vi "SEA_9811_Init.vi"(7 "Run?":bool=TRUE, 8 "error in":errorcluster, 9 "Transmit Channels Ref in":T1 format="%.0x", 10 "SEA9811_conf_cluster":T9={"FPGA resource name"="RIO0", "Rx ch conf (0..7)"=[{"Rx Channel Number (0..7)"=0, "Rx Label Filter"={"Label 00"=0, "Label 01"=0, "Label 02"=0, "Label 03"=0, "Label 04"=0, "Label 05"=0, "Label 06"=0, "Label 07"=0, "Label 08"=0, "Label 09"=0, "Label 10"=0, "Label 11"=0, "Label 12"=0, "Label 13"=0, "Label 14"=0, "Label 15"=0}, "Receiver Control Register (RCR)"={"RCR0: Data rate = ARINC 429 High-Speed (0) or Low-Speed (1)"=FALSE, "RCR1: not used"=FALSE, "RCR2: Label recognition for this channel enabled (1) or disabled (0)"=FALSE, "RCR3: Receiver channel disabled (1) or enabled (0)"=FALSE, "RCR4: Odd parity check for this channel enabled (1) or disabled (0"=FALSE, "RCR5: Receiver normal operation (1) or loopback mode (0)"=TRUE, "RCR6: Receiver Decoder disabled (0) or enabled (1) \n-> ARINC bits 10 and 9 must match RCR7 and RCR8"=FALSE, "RCR7: If receiver decoder is enabled (RCR6=1), \nthe ARINC bit 10 must match this bit"=FALSE, "RCR8: If receiver decoder is enabled (RCR6=1), \nthe ARINC bit 9 must match this bit"=FALSE, "RCR9: Label bit order for this channel non-reversed (1) \nor reversed (0)"=FALSE, "RCR10: not used"=FALSE, "RCR11: not used"=FALSE, "RCR12: not used"=FALSE, "RCR13: not used"=FALSE, "RCR14: not used"=FALSE, "RCR15: not used"=FALSE}}], "Transmitter Control Register (TCR)"={"TCR0: not used"=FALSE, "TCR1: not used"=FALSE, "TCR2: not used"=FALSE, "TCR3: Transmitter Parity Bit Enable: 32nd bit is parity (1) or data (0)"=FALSE, "TCR4: not used"=FALSE, "TCR5: not used"=FALSE, "TCR6: not used"=FALSE, "TCR7: not used"=FALSE, "TCR8: not used"=FALSE, "TCR9: Transmitter Parity Select: odd parity (0) or even parity (1)"=FALSE, "TCR10: Transmitter Data Rate: ARINC 429 high-speed (0) or low-speed (1)"=FALSE, "TCR11: ARINC Label Bit Order: label bit order reversed (0) or not reversed (1)"=FALSE, "TCR12: Disable Line Driver: normal operation (0) or transmitter disabled (1)"=FALSE, "TCR13: Tansmit whenever data is available in FIFO (1) or only start by instruction \"Enable Transmission\" (0)"=TRUE, "TCR14: not used"=FALSE, "TCR15: not used"=FALSE}, "Bitfile Path"=path ""}, 11 "Device Reference in":T1 format="%.0x") -> (0 "error out":errorcluster, 2 "SEA9811_RT_data out":T2 {"Tx"."Tx Refs (Data,Trig)"."Data Reference" format="%.0x"}, 3 "Device Reference out":T1 format="%.0x")   [LabVIEW 2015]
uses:
  Typdefs/SEA9811_RT_conf_cluster.ctl
  <vilib>/userdefined/High Color/nirio_resource_hc.ctl
  FPGA/SEA-9811_ReceiverAndTransmitter/SubVIs/SEA-9811_ReceiverAndTransmitter_RCR.ctl
  FPGA/SEA-9811_ReceiverAndTransmitter/SubVIs/SEA-9811_ReceiverAndTransmitter_TCR.ctl
  Typdefs/SEA9811_RT_data_cluster.ctl
  <userlib>/_FPGA Interface Advanced Tools/FPGA Interface Base/FPGA Interface Base.lvclass
  Typdefs/FPGA ref.ctl
  Typdefs/channel.ctl
  Typdefs/received word.ctl
  Typdefs/SEA9811_FPGA_FP_Addresses.ctl
  <vilib>/NI Veristand/Custom Device API/Block Data Reference.ctl
  <vilib>/NI Veristand/Custom Device API/Data Reference.ctl
  <vilib>/NI Veristand/Custom Device API/Custom Device Item Ref.ctl
  <vilib>/NI Veristand/Custom Device API/Data Access Type.ctl
  <vilib>/NI VeriStand/Custom Device API/Custom Device API.lvlib
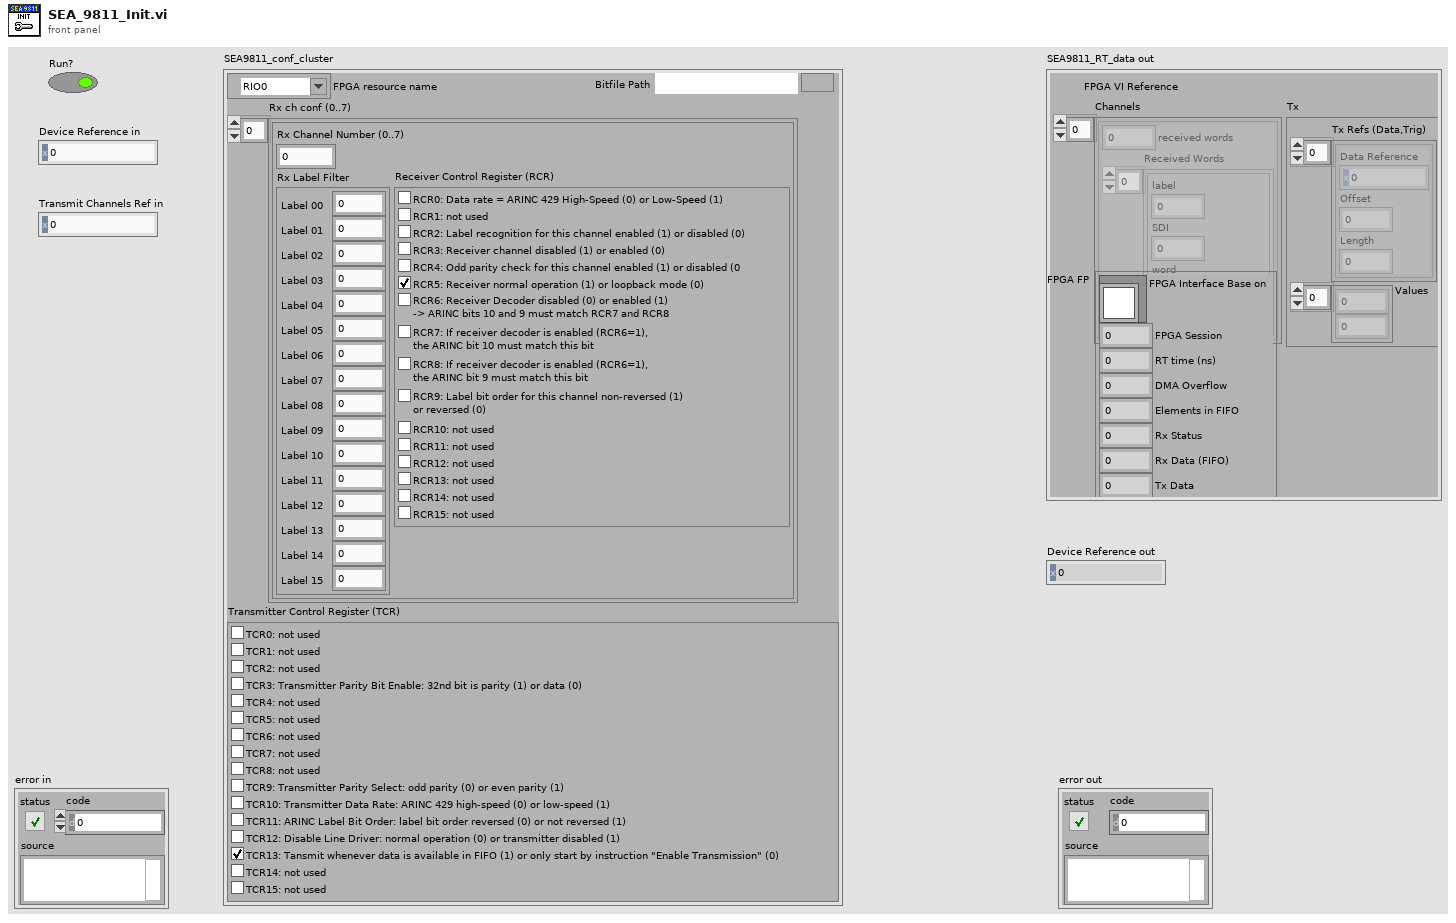
[diagram p1: front panel]
types:
  T1 = typedef "Custom Device API.lvlib/Custom Device Item Ref.ctl" = u64
  T2 = typedef "SEA9811_RT_data_cluster.ctl" = cluster{"FPGA VI Reference":T3, "Channels":T4[], "FPGA FP":T6, "Tx":cluster{"Tx Refs (Data,Trig)":T7[], "Values":dbl[]}}
  T3 = typedef "FPGA ref.ctl" = refnum<k20>
  T4 = typedef "channel.ctl" = cluster{"received words":u32, "Received Words":T5[]}
  T5 = typedef "received word.ctl" = cluster{"label":u8, "SDI":u8, "word":u32, "timestamp":dbl}
  T6 = typedef "SEA9811_FPGA_FP_Addresses.ctl" = cluster{"FPGA Interface Base on":refnum<class "FPGA Interface Base.lvclass">, "FPGA Session":u32, "RT time (ns)":u32, "DMA Overflow":u32, "Elements in FIFO":u32, "Rx Status":u32, "Rx Data (FIFO)":u32, "Tx Data":u32, "Transmit Data":u32}
  T7 = typedef "Custom Device API.lvlib/Block Data Reference.ctl" = cluster{"Data Reference":T8, "Offset":u64, "Length":u64}
  T8 = typedef "Custom Device API.lvlib/Data Reference.ctl" = i32
  T9 = typedef "SEA9811_RT_conf_cluster.ctl" = cluster{"FPGA resource name":T10, "Rx ch conf (0..7)":cluster{"Rx Channel Number (0..7)":u8, "Rx Label Filter":cluster{"Label 00":u8, "Label 01":u8, "Label 02":u8, "Label 03":u8, "Label 04":u8, "Label 05":u8, "Label 06":u8, "Label 07":u8, "Label 08":u8, "Label 09":u8, "Label 10":u8, "Label 11":u8, "Label 12":u8, "Label 13":u8, "Label 14":u8, "Label 15":u8}, "Receiver Control Register (RCR)":T11}[], "Transmitter Control Register (TCR)":T12, "Bitfile Path":path}
  T10 = typedef "nirio_resource_hc.ctl" = tag
  T11 = typedef "SEA-9811_ReceiverAndTransmitter_RCR.ctl" = cluster{"RCR0: Data rate = ARINC 429 High-Speed (0) or Low-Speed (1)":bool, "RCR1: not used":bool, "RCR2: Label recognition for this channel enabled (1) or disabled (0)":bool, "RCR3: Receiver channel disabled (1) or enabled (0)":bool, "RCR4: Odd parity check for this channel enabled (1) or disabled (0":bool, "RCR5: Receiver normal operation (1) or loopback mode (0)":bool, "RCR6: Receiver Decoder disabled (0) or enabled (1) \n-> ARINC bits 10 and 9 must match RCR7 and RCR8":bool, "RCR7: If receiver decoder is enabled (RCR6=1), \nthe ARINC bit 10 must match this bit":bool, "RCR8: If receiver decoder is enabled (RCR6=1), \nthe ARINC bit 9 must match this bit":bool, "RCR9: Label bit order for this channel non-reversed (1) \nor reversed (0)":bool, "RCR10: not used":bool, "RCR11: not used":bool, "RCR12: not used":bool, "RCR13: not used":bool, "RCR14: not used":bool, "RCR15: not used":bool}
  T12 = typedef "SEA-9811_ReceiverAndTransmitter_TCR.ctl" = cluster{"TCR0: not used":bool, "TCR1: not used":bool, "TCR2: not used":bool, "TCR3: Transmitter Parity Bit Enable: 32nd bit is parity (1) or data (0)":bool, "TCR4: not used":bool, "TCR5: not used":bool, "TCR6: not used":bool, "TCR7: not used":bool, "TCR8: not used":bool, "TCR9: Transmitter Parity Select: odd parity (0) or even parity (1)":bool, "TCR10: Transmitter Data Rate: ARINC 429 high-speed (0) or low-speed (1)":bool, "TCR11: ARINC Label Bit Order: label bit order reversed (0) or not reversed (1)":bool, "TCR12: Disable Line Driver: normal operation (0) or transmitter disabled (1)":bool, "TCR13: Tansmit whenever data is available in FIFO (1) or only start by instruction \"Enable Transmission\" (0)":bool, "TCR14: not used":bool, "TCR15: not used":bool}
  T13 = cluster{"Rx Channel Number (0..7)":u8, "Rx Label Filter":cluster{"Label 00":u8, "Label 01":u8, "Label 02":u8, "Label 03":u8, "Label 04":u8, "Label 05":u8, "Label 06":u8, "Label 07":u8, "Label 08":u8, "Label 09":u8, "Label 10":u8, "Label 11":u8, "Label 12":u8, "Label 13":u8, "Label 14":u8, "Label 15":u8}, "Receiver Control Register (RCR)":T11}[]
  T14 = typedef "Custom Device API.lvlib/Data Access Type.ctl" = enum16{"Read", "Write"}
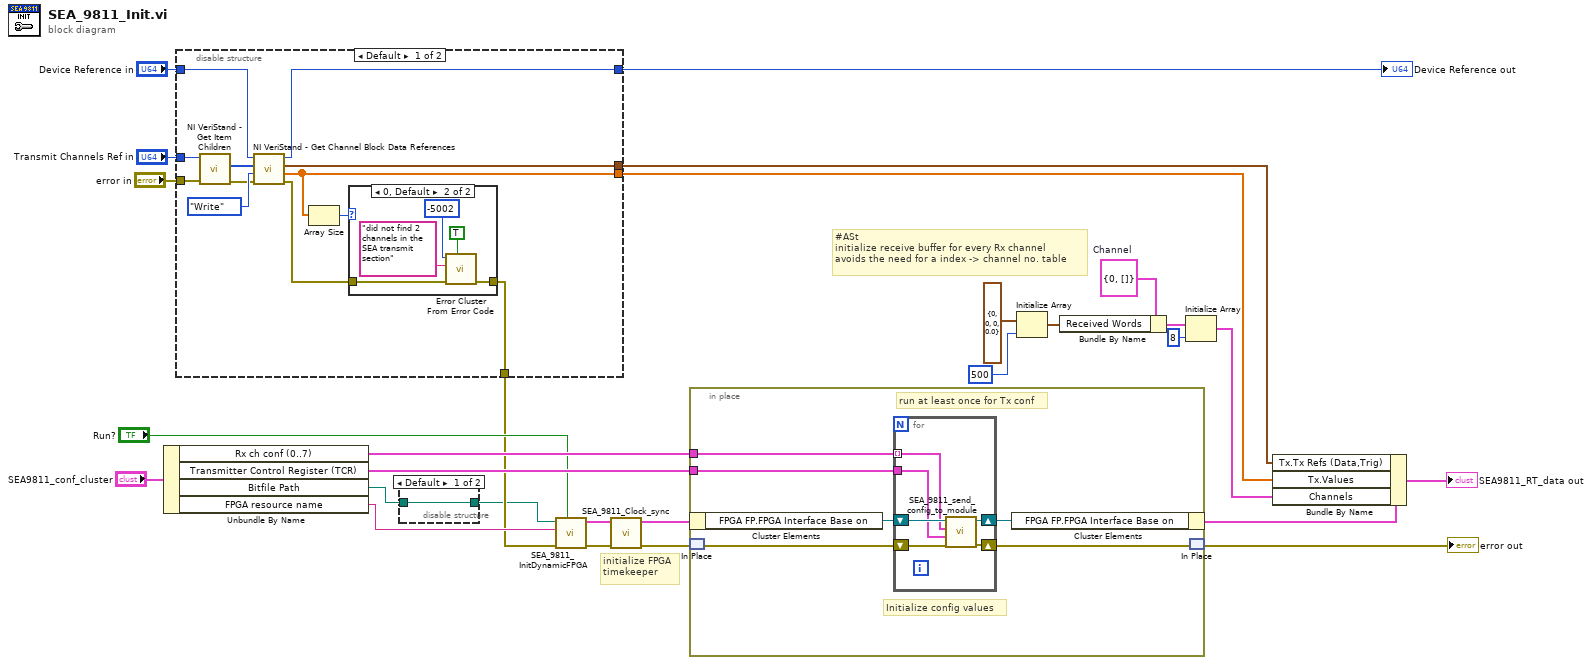
[diagram p0: block diagram]
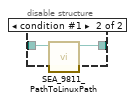
[diagram p2: hidden frame]
diagram:
  w22 = T4 {"received words"=0, "Received Words"=[]}  # Channel
  # "initialize FPGA\ntimekeeper"
  # "#ASt \ninitialize receive buffer for every Rx channel\navoids the need for a index -> channel no. table"
  n1 = Unbundle By Name("SEA9811_conf_cluster") -> ("Rx ch conf (0..7)"=w27:T13, "Transmitter Control Register (TCR)"=w26:T12, "Bitfile Path"=w2:path, "FPGA resource name"=w17:T10)
  n2 = disable-structure shown="Default" {
    disable-tunnel: "Transmit Channels Ref in" -> [w40 _]
    disable-tunnel: "Device Reference in" -> [w39 w48]
    disable-tunnel: [w38 w48] -> w7
    disable-tunnel: "error in" -> [w35 w47]
    disable-tunnel: [w34 w47] -> w5
    disable-tunnel: [w33 _] -> w4
    disable-tunnel: [w32 _] -> w3
    frame condition #0 (active) {
      n3 = call <vilib>:"NI VeriStand - Get Item Children.vi"("error in (no error)"=w35, "Item Ref in"=w40) -> ("error out"=w29:errorcluster, "Child Refs"=w31:T1[])  [unwired: 6 in, 2 out]
      n4 = call <vilib>:"NI VeriStand - Get Channel Block Data References.vi"("error in (no error)"=w29, "Access"=Data_Access_Type."Write", "Channel Refs"=w31, "Device Ref in"=w39) -> ("error out"=w36:errorcluster, "Values Array"=w33:dbl[], "Block Data Refs"=w32:T7[], "Device Ref out"=w38:T1)  [unwired: 4 in]
      n5 = Array Size(array=w33) -> (size(s)=w37:i32)
      n6 = case shown="0, Default" w37 {
        tunnel: w36 -> [w41 w44]
        tunnel: [w41 w43] -> w34
        frame 2 {
        }
        frame 0, Default {
          n7 = call <vilib>:"Error Cluster From Error Code.vi"("show call chain? (False)"=TRUE, "error in (no error)"=w44, "error message (\"\")"="did not find 2 channels in the SEA transmit section" ("error message (\"\")"), "error code (0)"=-5002) -> ("error out"=w43:errorcluster)  [unwired: 5 in]
        }
      }
    }
    frame condition #1 {
    }
  }
  "Device Reference out" <- w7
  n8 = disable-structure shown="Default" {
    disable-tunnel: w2 -> [w49 w51]
    disable-tunnel: [w49 w50] -> w1
    frame condition #0 (active) {
    }
    frame condition #1 {
      n9 = call "SEA_9811_PathToLinuxPath.vi"("Path in"=w51) -> ("Path out"=w50:path)  [unwired: 10 in]
    }
  }
  n10 = call "SEA_9811_InitDynamicFPGA.vi"("Run?"="Run?", "error in (no error)"=w5, "FPGA resource name"=w17, "Bitfile Path"=w1) -> ("error out"=w11:errorcluster, "SEA9811_RT_data out"=w13:T2)  [unwired: 6 in]
  n11 = call "SEA_9811_Clock_sync.vi"("error in (no error)"=w11, "SEA9811_RT_data in"=w13) -> ("error out"=w10:errorcluster, "SEA9811_RT_data out"=w12:T2)  [unwired: 8 in]
  n12 = in-place {
    in-place-border: w27 -> [w57]
    in-place-border: w26 -> [w56]
    # "run at least once for Tx conf"
    # "Initialize config values"
    n13 = in-place-cluster #1(w12) -> ("FPGA FP.FPGA Interface Base on"=w53:refnum<class "FPGA Interface Base.lvclass">)
    n14 = in-place-match #2(w10) -> (w54:errorcluster)
    n15 = for {
      shift-right: [w60] -> w55
      shift-left: w54 -> [w62]
      shift-right: [w61] -> w52
      shift-left: w53 -> [w63]
      tunnel: w57 -> [w59] mode=indexing
      tunnel: w56 -> [w58]
      n16 = call "SEA_9811_send_config_to_module.vi"("error in (no error)"=w62, "Transmitter Control Register (TCR)"=w58, "Rx channel"=w59, "FPGA Interface Base In"=w63) -> ("error out"=w60:errorcluster, "FPGA Interface Base Out"=w61:refnum<class "FPGA Interface Base.lvclass">)  [unwired: 6 in]
    }
    n17 = in-place-cluster #1("FPGA FP.FPGA Interface Base on"=w52) -> (w14:T2)
    n18 = in-place-match #2(w55) -> (→"error out":errorcluster)
  }
  n19 = Initialize Array(T5 {"label"=0, "SDI"=0, "word"=0, "timestamp"=0.0} ("received word"), 500 ("dimension size")) -> (w21:T5[])
  n20 = Bundle By Name(cluster=w22, "Received Words"=w21) -> (w20:T4)
  n21 = Initialize Array(w20, 8 ("dimension size")) -> (w18:T4[])
  n22 = Bundle By Name(cluster=w14, "Tx.Tx Refs (Data,Trig)"=w3, "Tx.Values"=w4, "Channels"=w18) -> (→"SEA9811_RT_data out":T2)
